vi "moving forward.vi"(0 "time?":bool, 4 "kp+ right":T4, 5 "Delay (s)":dbl, 6 "kp+ left":T1, 7 "cm":dbl, 8 "kp- right":T2, 9 "kp- left":T3, 10 "maxspeed":dbl) -> ()   [LabVIEW 2016]
uses:
  Control 4.ctl
  Control 2.ctl
  Control 1.ctl
  Control 3.ctl
  <vilib>/Rock Robotics/WPI/Utilities/WPI_GetSetVariantRefNum.vi
  distance to target.vi
panel:
  out "Boolean":bool
  in  "right":dbl
  out "pi":dbl
  out "angle 2":dbl
  out "distance to target 4":dbl
  out "angle":dbl=360.0
  in  "Feed time (s)":dbl=0.05
  in  "left":dbl
  in  "startspeed":dbl
  in  "time":dbl
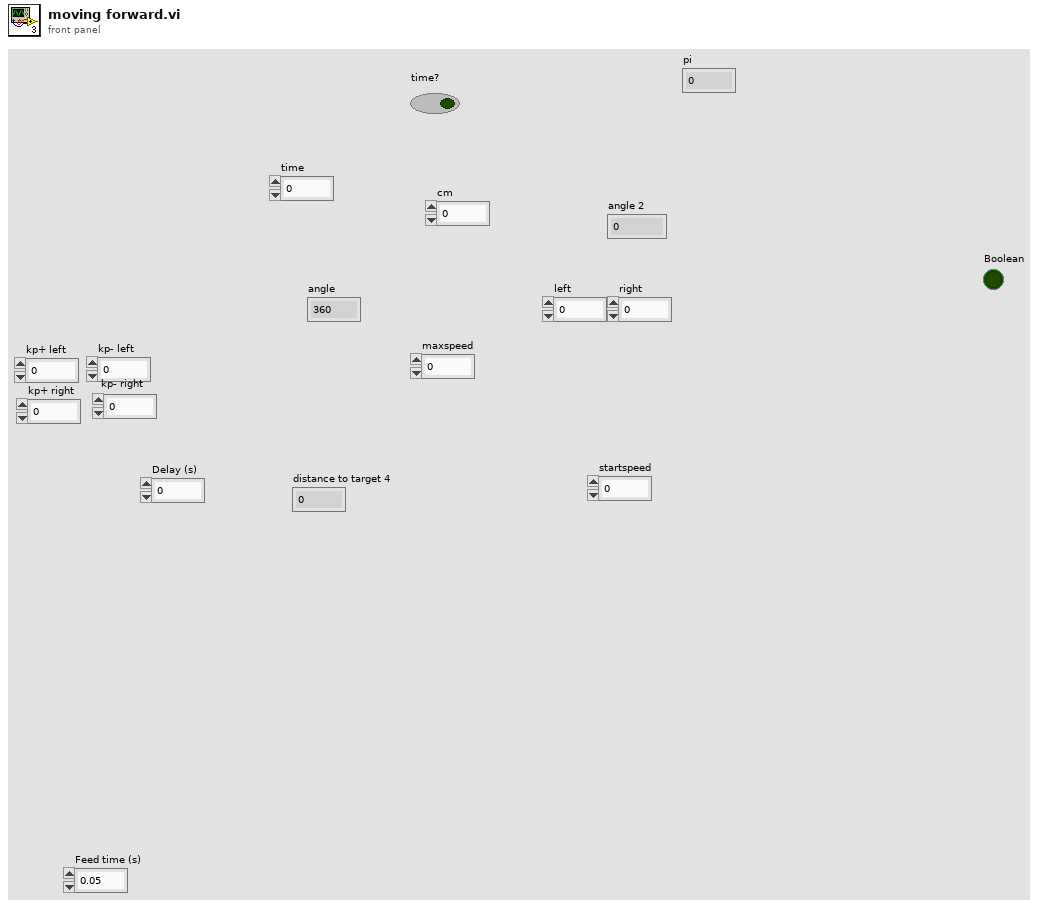
[diagram p1: front panel]
types:
  T1 = typedef "Control 3.ctl" = dbl
  T2 = typedef "Control 1.ctl" = dbl
  T3 = typedef "Control 2.ctl" = dbl
  T4 = typedef "Control 4.ctl" = dbl
  T5 = typedef "WPI_GyroDevRef.ctl" = cluster{"DevStatus":errorcluster, "Analog Channel":T6, "Offset":dbl, "Gain (VoltsPerDegree/Second)":dbl, "Gyro Type":enum16{"Analog", "XRS450"}, "Handle":i32, "SPI Bus":T7, "Device Found":bool, "Sample Rate":dbl, "Calibrate On Open":bool}
  T6 = typedef "FPGA_AIChannel.ctl" = enum8{"AI 0", "AI 1", "AI 2", "AI 3", "AI MXP 0", "AI MXP 1", "AI MXP 2", "AI MXP 3", "Invalid"}
  T7 = typedef "spi_bus.ctl" = enum16{"SPI On-Board, CS0", "SPI On-Board, CS1", "SPI On-Board, CS2", "SPI On-Board, CS3", "SPI MXP", "Invalid"}
  T8 = typedef "WPI_RobotDriveDevRef.ctl" = cluster{"DevStatus":errorcluster, "Motors[]":T9[], "Square Inputs":bool, "Max Output":dbl}
  T9 = typedef "WPI_MotorControlDeviceRef.ctl" = cluster{"DeviceStatus":errorcluster, "Type":T10, "PWM":cluster{"PWM Channel":T11, "DeadBand":T12}, "CAN":cluster{"Device Number":u8, "SetOutput VI Ref":variant, "GetOutput VI Ref":variant, "Enable VI Ref":variant, "Disable VI Ref":variant, "Data":variant}, "Invert":bool}
  T10 = typedef "WPI_MotorControlType.ctl" = enum16{"PWM", "CAN"}
  T11 = typedef "FPGA_DIOPWMChannel.ctl" = enum8{"PWM 0", "PWM 1", "PWM 2", "PWM 3", "PWM 4", "PWM 5", "PWM 6", "PWM 7", "PWM 8", "PWM 9", "PWM MXP 0", "PWM MXP 1", "PWM MXP 2", "PWM MXP 3", "PWM MXP 4", "PWM MXP 5", "PWM MXP 6", "PWM MXP 7", "PWM MXP 8", "PWM MXP 9", "Invalid"}
  T12 = typedef "WPI_PWMDeadband.ctl" = cluster{"Name":string, "maxPositivePwm":i32, "minPositivePwm":i32, "centerPwm":i32, "maxNegativePwm":i32, "minNegativePwm":i32, "angularRange":u16}
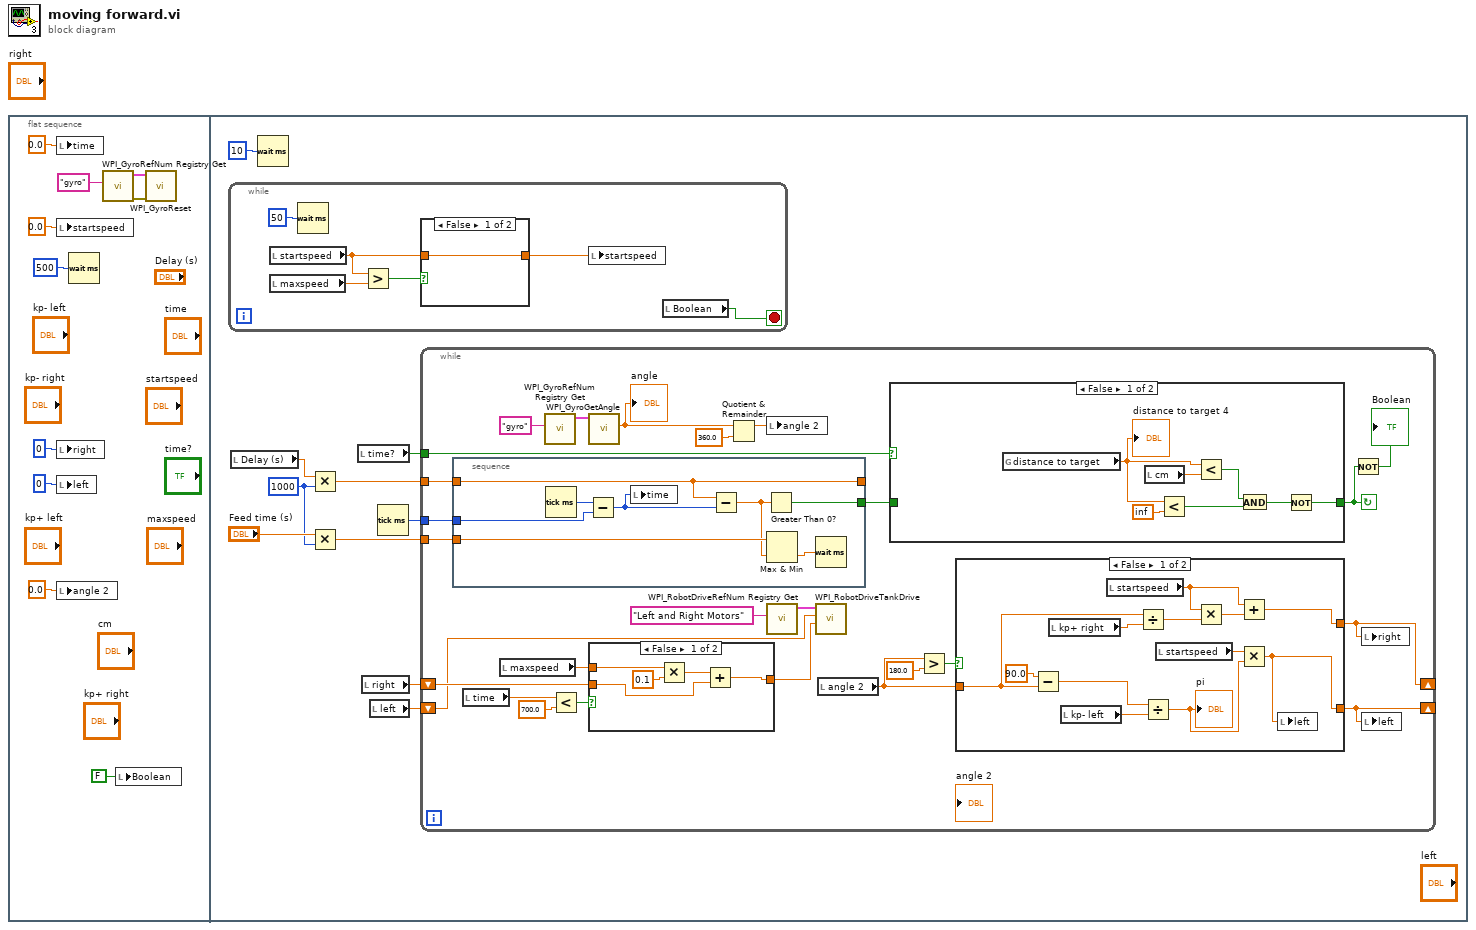
[diagram p0: block diagram]
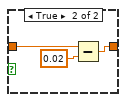
[diagram p2: hidden frame]
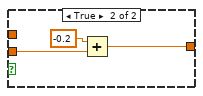
[diagram p4: hidden frame]
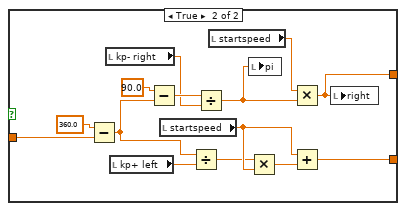
[diagram p5: hidden frame]
diagram:
  n1 = flat-sequence {
    frame #0 {
      n2 = local write "time"(0.0 ("time")) -> ()
      n3 = local write "startspeed"(0.0 ("startspeed")) -> ()
      n4 = local write "right"(0) -> ()
      n5 = local write "left"(0) -> ()
      n6 = local write "angle 2"(0.0 ("angle")) -> ()
      n7 = Wait (ms)(milliseconds to wait=u32 500) -> ()  [unwired: 1 out]
      n8 = call <vilib>:"WPI_GyroRefNum Registry Get.vi"("refnum name"="gyro") -> ("error out"=w8:errorcluster, "GyroDevRef"=w9:T5)  [unwired: 9 in]
      n9 = local write "Boolean"(FALSE ("Boolean")) -> ()
      n10 = call <vilib>:"WPI_GyroReset.vi"("error in"=w8, "GyroDevRef"=w9) -> ()  [unwired: 8 in, 2 out]
    }
    frame #1 {
      w19 = 1000
      n11 = while {
        stop <- w21 stop-if-true
        n12 = local read "startspeed"() -> (w23:dbl)
        n13 = local read "maxspeed"() -> (w22:dbl)
        n14 = Wait (ms)(milliseconds to wait=u32 50) -> ()  [unwired: 1 out]
        n15 = Greater?(x=w23, y=w22) -> (0:w24:bool)
        n16 = case shown="False" w24 {
          tunnel: w23 -> [w27 w30]
          tunnel: [w27 w29] -> w25
          frame False {
          }
          frame True {
            n17 = Subtract(x=w30, y=0.02) -> (x-y=w29:dbl)
          }
        }
        n18 = local write "startspeed"(w25) -> ()
        n19 = local read "Boolean"() -> (w21:bool)
      }
      n20 = local read "Delay (s)"() -> (w11:dbl)
      n21 = Wait (ms)(milliseconds to wait=u32 10) -> ()  [unwired: 1 out]
      n22 = Multiply(x=w11, y=w19) -> (x*y=w17:dbl)
      n23 = Multiply(x="Feed time (s)", y=w19) -> (x*y=w18:dbl)
      n24 = local read "time?"() -> (w12:bool)
      n25 = local read "right"() -> (w14:dbl)
      n26 = local read "left"() -> (w15:dbl)
      n27 = Tick Count (ms)() -> (millisecond timer value=w16:u32)
      n28 = while {
        tunnel: w17 -> [w37]
        tunnel: w18 -> [w35]
        tunnel: w16 -> [w36]
        shift-right: [w46] -> _
        shift-left: w14 -> [w42]
        shift-right: [w47] -> _
        shift-left: w15 -> [w40]
        tunnel: w12 -> [w38]
        stop <- w31 continue-if-true
        n29 = stacked-sequence {
          tunnel: w36 -> [w64]
          tunnel: w35 -> [w63]
          tunnel: [w57] -> _
          tunnel: [w60] -> w34
          tunnel: w37 -> [w57]
          frame #0 {
            n30 = Tick Count (ms)() -> (millisecond timer value=w61:u32)
            n31 = Subtract(x=w61, y=w64) -> (x-y=w58:u32)
            n32 = local write "time"(w58) -> ()
            n33 = Subtract(x=w57, y=w58) -> (x-y=w59:dbl)
            n34 = Greater Than 0?(x=w59) -> (x > 0?=w60:bool)
            n35 = Max & Min(x=w63, y=w59) -> (min(x,y)=w62:dbl)  [unwired: 1 out]
            n36 = Wait (ms)(milliseconds to wait=w62) -> ()  [unwired: 1 out]
          }
        }
        n37 = local read "time"() -> (w44:dbl)
        n38 = local read "maxspeed"() -> (w33:dbl)
        n39 = call <vilib>:"WPI_GyroRefNum Registry Get.vi"("refnum name"="gyro") -> ("GyroDevRef"=w54:T5)  [unwired: 9 in, 1 out]
        n40 = Less?(x=w44, y=700.0) -> (x < y?=w45:bool)
        n41 = call <vilib>:"WPI_GyroGetAngle.vi"("GyroDevRef"=w54) -> ("Angle"=w39:dbl)  [unwired: 6 in, 4 out]
        "angle" <- w39
        n42 = case shown="False" w45 {
          tunnel: [w76 w79] -> w41
          tunnel: w42 -> [w77 w78]
          tunnel: w33 -> [w74 _]
          frame False {
            n43 = Multiply(x=w74, y=0.1) -> (x*y=w75:dbl)
            n44 = Add(x=w75, y=w77) -> (x+y=w76:T2)
          }
          frame True {
            n45 = Add(x=-0.2, y=w78) -> (x+y=w79:T2)
          }
        }
        n46 = Quotient & Remainder(x=w39, y=360.0) -> (x-y*floor(x/y)=w51:dbl)  [unwired: 1 out]
        n47 = local write "angle 2"(w51) -> ()
        n48 = call <vilib>:"WPI_RobotDriveRefNum Registry Get.vi"("refnum name"="Left and Right Motors") -> ("RobotDriveDevRef"=w56:T8)  [unwired: 1 in, 9 out]
        n49 = call <vilib>:"WPI_RobotDriveTankDrive.vi"("Right axis value"=w41, "Left axis value"=w40, "RobotDriveDevRef"=w56) -> ()  [unwired: 6 in, 3 out]
        n50 = local read "angle 2"() -> (w48:dbl)
        n51 = case shown="False" w38 {
          tunnel: [w65 w72] -> w31
          tunnel: w34 -> [_ w72]
          frame False {
            n52 = global read "distance to target.vi" "distance to target"() -> (w70:dbl)
            "distance to target 4" <- w70
            n53 = local read "cm"() -> (w69:dbl)
            n54 = Less?(x=w70, y=inf) -> (x < y?=w67:bool)
            n55 = Less?(x=w70, y=w69) -> (x < y?=w68:bool)
            n56 = And(x=w68, y=w67) -> (x .and. y?=w66:bool)
            n57 = Not(x=w66) -> (.not. x?=w65:bool)
          }
          frame True {
          }
        }
        n58 = Greater?(x=w48, y=180.0) -> (0:w49:bool)
        n59 = case shown="False" w49 {
          tunnel: w48 -> [w83 w104]
          tunnel: [w89 w103] -> w46
          tunnel: [w91 w100] -> w47
          frame False {
            n60 = Subtract(x=90.0, y=w83) -> (x-y=w85:dbl)
            n61 = local read "kp+ right"() -> (w82:T4)
            n62 = local read "kp- left"() -> (w81:T3)
            n63 = local read "startspeed"() -> (w87:dbl)
            n64 = Divide(x=w83, y=w82) -> (x/y=w84:T4)
            n65 = Divide(x=w85, y=w81) -> (x/y=w86:T3)
            "pi" <- w86
            n66 = local read "startspeed"() -> (w92:dbl)
            n67 = Multiply(x=w87, y=w84) -> (x*y=w88:T4)
            n68 = Add(x=w87, y=w88) -> (x+y=w89:T4)
            n69 = Multiply(x=w92, y=w86) -> (x*y=w91:T3)
            n70 = local write "left"(w91) -> ()
          }
          frame True {
            n71 = Subtract(x=360.0, y=w104) -> (x-y=w95:dbl)
            n72 = local read "kp- right"() -> (w93:T2)
            n73 = local read "kp+ left"() -> (w94:T1)
            n74 = Subtract(x=90.0, y=w95) -> (x-y=w97:dbl)
            n75 = local read "startspeed"() -> (w98:dbl)
            n76 = Divide(x=w95, y=w94) -> (x/y=w96:T1)
            n77 = Divide(x=w97, y=w93) -> (x/y=w101:T2)
            n78 = local read "startspeed"() -> (w106:dbl)
            n79 = local write "pi"(w101) -> ()
            n80 = Multiply(x=w96, y=w98) -> (x*y=w99:T1)
            n81 = Multiply(x=w106, y=w101) -> (x*y=w103:T2)
            n82 = Add(x=w98, y=w99) -> (x+y=w100:T1)
            n83 = local write "right"(w103) -> ()
          }
        }
        n84 = Not(x=w31) -> (.not. x?=→"Boolean":bool)
        n85 = local write "right"(w46) -> ()
        n86 = local write "left"(w47) -> ()
      }
    }
  }
